vi "Get Current Control Values.vi"(8 "error in":errorcluster, 10 "Humidifier":string="med", 11 "Controller in":refnum<class "Controller.lvclass">) -> (0 "error out":errorcluster, 1 "Ctl":bool, 2 "Control values":T1, 3 "Controller Out":refnum<class "Controller.lvclass">)   [LabVIEW 2014, in "Controller.lvlib" / "Controller.lvclass"]
uses:
  Controller.lvclass
  reusable/Session APIs/CVT/CVT.lvclass
  reusable/Session APIs/Session Log/System Log.lvclass
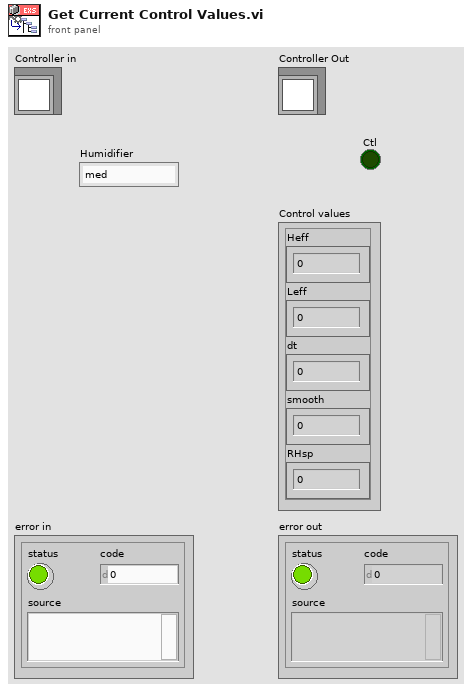
[diagram p1: front panel]
types:
  T1 = cluster{"Heff":dbl, "Leff":dbl, "dt":dbl, "smooth":dbl, "RHsp":dbl}
  T2 = typedef "Session - Root.lvclass/Session Handle.ctl" = refnum<data-value>
  T3 = cluster{"[0]":dbl, "[1]":dbl, "[2]":dbl, "[3]":dbl, "[4]":dbl}
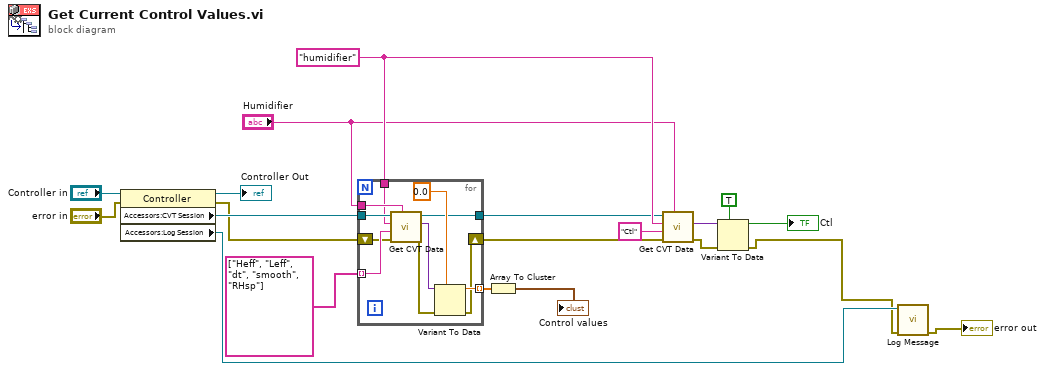
[diagram p0: block diagram]
diagram:
  w19 = "humidifier" ("Group")
  n1 = property class="Controller"(reference="Controller in", error in="error in") -> (reference out=→"Controller Out":refnum<class "Controller.lvclass">, error out=w13:errorcluster, "Accessors:CVT Session"=w14:T2, "Accessors:Log Session"=w11:T2)
  n2 = for {
    tunnel: w14 -> [w31]
    tunnel: "Humidifier" -> [w30]
    tunnel: string[] ["Heff", "Leff", "dt", "smooth", "RHsp"] ("Array 3") -> [w29] mode=indexing
    tunnel: w19 -> [w28]
    tunnel: [w25] -> w8 mode=indexing
    tunnel: [w24] -> w3
    shift-right: [w22] -> w2
    shift-left: w13 -> [w23]
    n3 = call "Get CVT Data.vi"("Subgroup"=w30, "error in"=w23, "Variable"=w29, "Group"=w28, "CVT Session In"=w31) -> ("error out"=w21:errorcluster, "Data Out"=w27:variant, "CVT Session Out"=w24:T2)  [unwired: 3 in, 1 out]
    n4 = Variant To Data(error in=w21, type=0.0, Variant=w27) -> (data=w25:dbl, error out=w22:errorcluster)
  }
  n5 = Array To Cluster(array=w8) -> (cluster=→"Control values":T3)
  n6 = call "Get CVT Data.vi"("Subgroup"="Humidifier", "error in"=w2, "Variable"="Ctl" ("string"), "Group"=w19, "CVT Session In"=w3) -> ("error out"=w4:errorcluster, "Data Out"=w6:variant)  [unwired: 3 in, 2 out]
  n7 = Variant To Data(error in=w4, type=TRUE, Variant=w6) -> (data=→"Ctl":bool, error out=w10:errorcluster)
  n8 = call "Log Message.vi"("error in"=w10, "session in"=w11) -> ("error out"=→"error out":errorcluster)  [unwired: 8 in, 1 out]
